vi "DLMoveAxis-Com-Exec.vi"(6 "ControlQueue":refnum<queue>, 7 "data":variant, 8 "error in (no error)":errorcluster, 9 "axisInum":refnum<vi>, 10 "AxisI":refnum<vi>, 11 "DelayLine in":refnum<class "DelayLine.lvclass">) -> (0 "error out":errorcluster, 3 "DelayLine out":refnum<class "DelayLine.lvclass">)   [LabVIEW 2015, in "DelayLine.lvclass"]
uses:
  DelayLine.lvclass
  dependecies/ControlsVIs/Clusters-def/DLMovedAxis-Com.ctl
  dependecies/ControlsVIs/Clusters-def/DL-Com-MoveAxis.ctl
  dependecies/ControlsVIs/Clusters-def/SERVER-Commands.ctl
  GeneralFunctionality/GeneralFunctionality.lvclass/GeneralFunctionality.ctl
  Control/Control-Server/Control-Server.lvclass
  GeneralFunctionality/GeneralFunctionality.lvclass
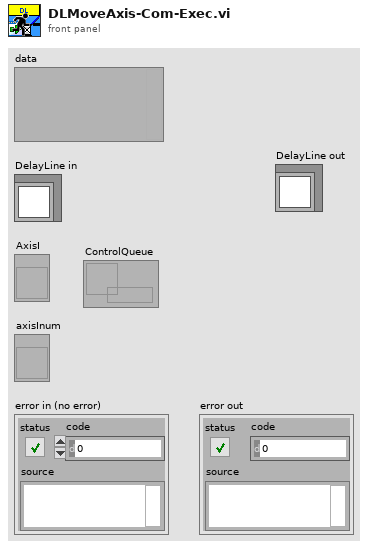
[diagram p1: front panel]
types:
  T1 = typedef "Control-Server.lvclass/SERVER-Commands.ctl" = string
  T2 = typedef "DelayLine.lvclass/DL-Com-MoveAxis.ctl" = cluster{"Axis":i32, "Where":dbl, "How":u16}
  T3 = typedef "DelayLine.lvclass/DLMovedAxis-Com.ctl" = cluster{"axis":i32, "what was asked":dbl, "where is is now":dbl, "Moved":bool, "error in (no error)":errorcluster}
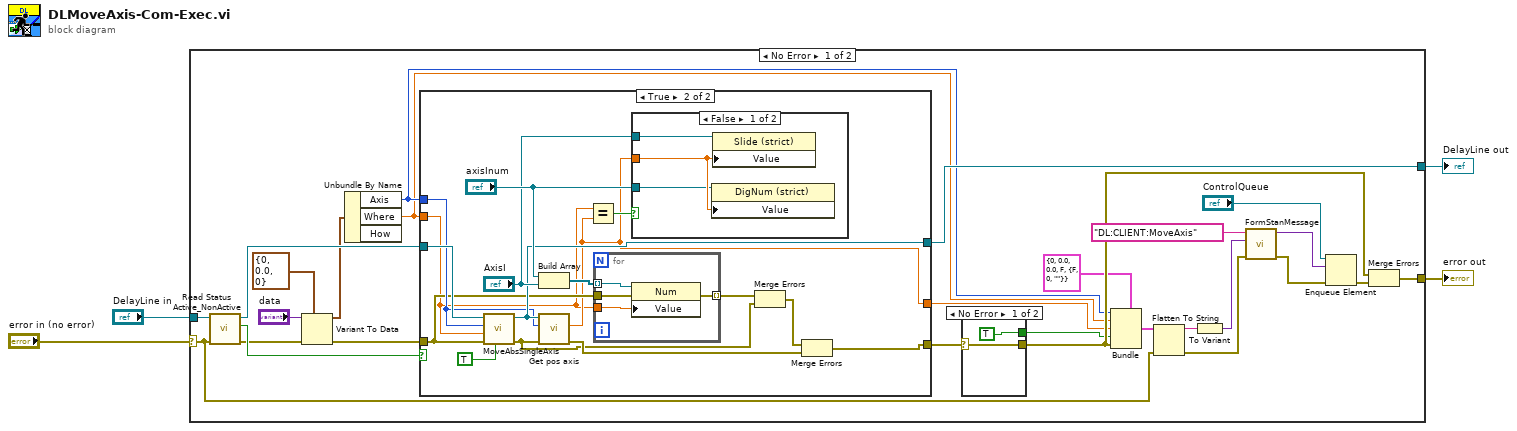
[diagram p0: block diagram]
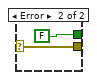
[diagram p2: hidden frame]
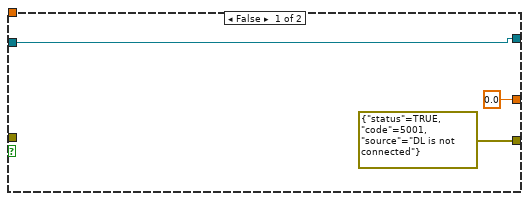
[diagram p3: hidden frame]
diagram:
  n1 = case shown="No Error" "error in (no error)" {
    selector: "error in (no error)" -> [w19 w62]
    tunnel: "DelayLine in" -> [w30 w63]
    tunnel: [w18 w62] -> w1
    tunnel: [w28 w63] -> w3
    frame No Error {
      n2 = call "Read Status Active_NonActive.vi"("error in (no error)"=w19, "GeneralFunctionality in"=w30) -> ("error out"=w15:errorcluster, "Status Active/NonActive"=w29:bool, "GeneralFunctionality out"=w31:refnum<class "DelayLine.lvclass">)  [unwired: 7 in]
      n3 = Variant To Data(error in=w15, type=T2 {"Axis"=0, "Where"=0.0, "How"=0} ("output cluster"), Variant="data") -> (data=w13:T2, error out=w14:errorcluster)
      n4 = Unbundle By Name(w13) -> ("Axis"=w12:i32, "Where"=w11:dbl)  [unwired: 1 out]
      n5 = case shown="True" w29 {
        tunnel: [w38 w46] -> w28
        tunnel: [errorcluster {"status"=TRUE, "code"=5001, "source"="DL is not connected"} ("error IO") w44] -> w20
        tunnel: w14 -> [_ w41]
        tunnel: w31 -> [w38 w43]
        tunnel: w12 -> [_ w42]
        tunnel: w11 -> [_ w39]
        tunnel: [0.0 ("Pos") w40] -> w10
        frame False {
        }
        frame True {
          n6 = call-dynamic "MoveAbsSingleAxis.vi"("Wait"=TRUE, "error in (no error)"=w41, "Value"=w39, "Axis"=w42, "DelayLine in"=w43) -> ("error out"=w47:errorcluster, "DelayLine out"=w46:refnum<class "DelayLine.lvclass">)  [unwired: 5 in]
          n7 = Build Array("axisInum", "AxisI") -> (w53:refnum<vi>[])
          n8 = call-dynamic "Get pos axis.vi"("error in (no error)"=w47, "Axis"=w42, "DelayLine in"=w46) -> ("error out"=w51:errorcluster, "Pos"=w40:dbl)  [unwired: 6 in, 1 out]
          n9 = Equal?(x=w39, y=w40) -> (x = y?=w50:bool)
          n10 = for {
            tunnel: w53 -> [w61] mode=indexing
            tunnel: w41 -> [w60]
            tunnel: [w59] -> w52 mode=indexing
            tunnel: w39 -> [w58]
            n11 = property class="Num"(reference=w61, error in=w60, "Value"=w58) -> (error out=w59:errorcluster)  [unwired: 1 out]
          }
          n12 = case shown="False" w50 {
            tunnel: w40 -> [w57 _]
            tunnel: "axisInum" -> [w56 _]
            tunnel: "AxisI" -> [w55 _]
            frame False {
              n13 = property class="DigNum (strict)"(reference=w56, "Value"=w57) -> ()  [unwired: 1 in, 2 out]
              n14 = property class="Slide (strict)"(reference=w55, "Value"=w57) -> ()  [unwired: 1 in, 2 out]
            }
            frame True {
            }
          }
          n15 = Merge Errors(w52, w47) -> (w45:errorcluster)
          n16 = Merge Errors(w45, w51) -> (w44:errorcluster)
        }
      }
      n17 = case shown="No Error" w20 {
        selector: w20 -> [w32 w34]
        tunnel: [TRUE FALSE] -> w24
        tunnel: [w32 w34] -> w25
        frame No Error {
        }
        frame Error {
        }
      }
      n18 = Bundle(cluster=T3 {"axis"=0, "what was asked"=0.0, "where is is now"=0.0, "Moved"=FALSE, "error in (no error)"={"status"=FALSE, "code"=0, "source"=""}}, "axis"=w12, "what was asked"=w11, "where is is now"=w10, "Moved"=w24, "error in (no error)"=w25) -> (w21:T3)
      n19 = Flatten To String(anything=w21, error in (no error)=w19) -> (data string=w22:string, error out=w9:errorcluster)  [unwired: 2 in, 1 out]
      n20 = To Variant(anything=w22) -> (Variant=w6:variant)
      n21 = call "FormStanMessage.vi"("error in"=w9, "data"=w6, "Command"=T1 "DL:CLIENT:MoveAxis" ("Commands")) -> ("error out"=w8:errorcluster, "message"=w7:variant)  [unwired: 7 in]
      n22 = Enqueue Element(queue="ControlQueue", element=w7, error in (no error)=w8) -> (error out=w27:errorcluster)  [unwired: 1 in, 2 out]
      n23 = Merge Errors(w25, w27) -> (w18:errorcluster)
    }
    frame Error {
    }
  }
  "error out" <- w1
  "DelayLine out" <- w3
